vi "Find Test Parameter Names.vi"(11 "Worksheet Data":string[][](array[string])) -> (1 "Test Parameter Row Index":i32, 2 "Test Parameters":string[](array[string]), 3 "Worksheet Data Out":string[][](array[string]))   [LabVIEW 2016, in "QPA TCF Parser.lvlib" / "QPA TCF Parser.lvclass"]
uses:
  QPA TCF Parser.lvclass
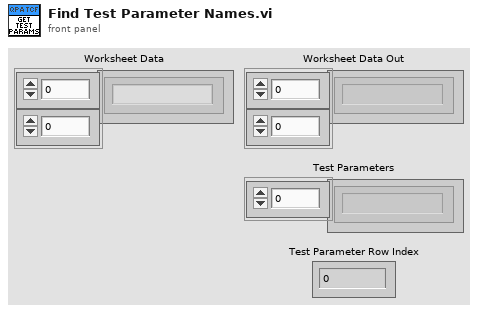
[diagram p1: front panel]
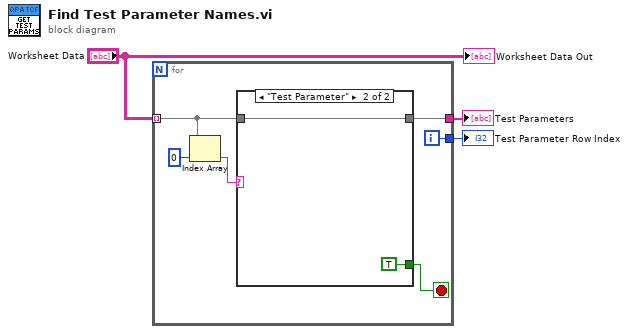
[diagram p0: block diagram]
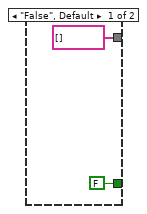
[diagram p2: hidden frame]
diagram:
  n1 = for {
    tunnel: "Worksheet Data" -> [w6] mode=indexing
    tunnel: [w5] -> w2
    tunnel: [w4] -> w1
    i -> [w4]
    stop <- w7 stop-if-true
    n2 = Index Array(array=w6, index=0) -> (element=w8:string)
    n3 = case shown="\"Test Parameter\"" w8 {
      tunnel: [FALSE TRUE] -> w7
      tunnel: [string[] [] ("Worksheet Data") w12] -> w5
      tunnel: w6 -> [_ w12]
      frame "False", Default {
      }
      frame "Test Parameter" {
      }
    }
  }
  "Test Parameters" <- w2
  "Test Parameter Row Index" <- w1
  "Worksheet Data Out" <- "Worksheet Data"
